vi "save.vi"(8 "error in (no error)":errorcluster, 11 "ScriptEditorV2 in":refnum<class "ScriptEditorV2.lvclass">) -> (0 "error out":errorcluster, 3 "ScriptEditorV2 out":refnum<class "ScriptEditorV2.lvclass">)   [LabVIEW 2009, in "Views.lvlib" / "ScriptEditor.lvlib" / "ScriptEditorV2.lvclass"]
uses:
  ScriptEditorV2.lvclass
  ScriptEditorV2.lvclass/ScriptEditorV2.ctl
  Tools/Scripting/DataPointScript/DataPointScript.lvclass
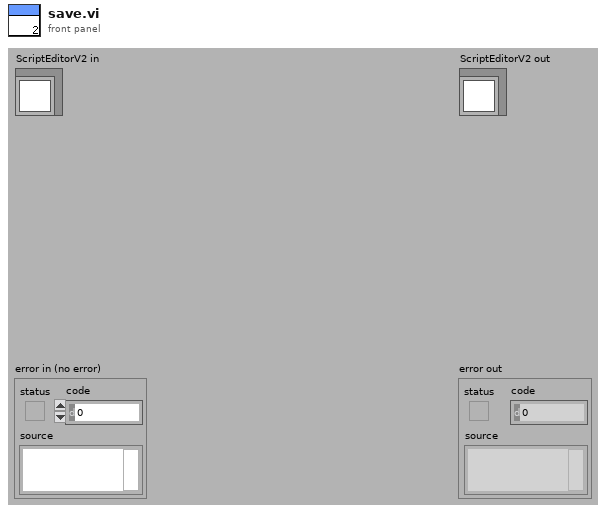
[diagram p1: front panel]
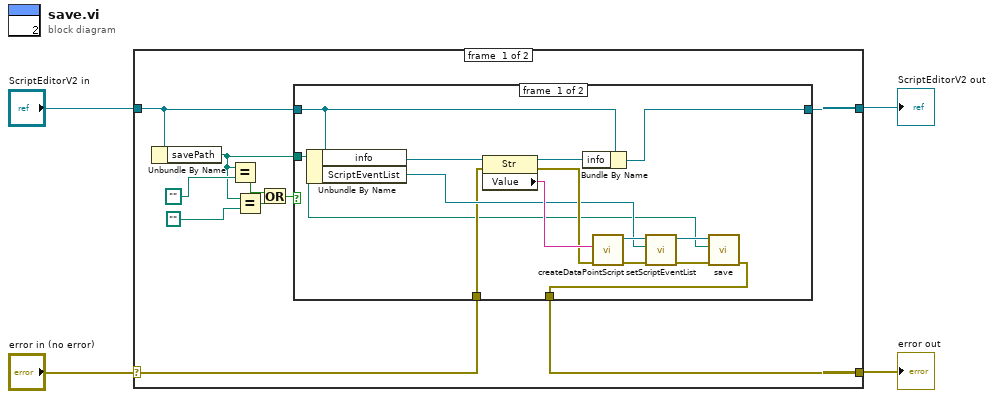
[diagram p0: block diagram]
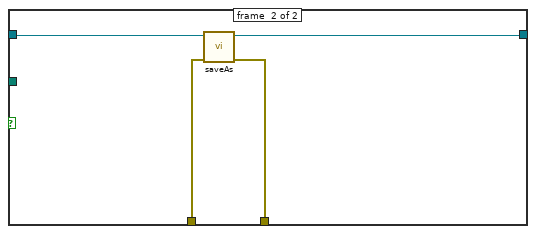
[diagram p2: hidden frame]
diagram:
  n1 = case shown="No Error" "error in (no error)" {
    selector: "error in (no error)" -> [w12 w34]
    tunnel: [w13 w34] -> w3
    tunnel: [w14 w33] -> w1
    tunnel: "ScriptEditorV2 in" -> [w11 w33]
    frame #0 {
      n2 = Unbundle By Name(w11) -> ("savePath"=w5:path)
      n3 = Equal?(x=w5, y=path "") -> (x = y?=w10:bool)
      n4 = Equal?(x=w5, y=path "") -> (x = y?=w7:bool)
      n5 = Or(x=w10, y=w7) -> (x .or. y?=w6:bool)
      n6 = case shown="False" w6 {
        tunnel: w11 -> [w24 w32]
        tunnel: [w23 w29] -> w14
        tunnel: [w17 w30] -> w13
        tunnel: w12 -> [w16 w31]
        tunnel: w5 -> [w15 _]
        frame #0 {
          n7 = Unbundle By Name(w24) -> ("info"=w28:refnum<vi>, "ScriptEventList"=w20:refnum<class "ScriptEventList.lvclass">)
          n8 = property class="Str"(reference=w28, error in=w16) -> (reference out=w25:refnum<vi>, error out=w26:errorcluster, "Value"=w27:string)
          n9 = Bundle By Name(cluster=w24, "info"=w25) -> (w23:refnum<class "ScriptEditorV2.lvclass">)
          n10 = call "createDataPointScript.vi"("error in (no error)"=w26, "script_comment"=w27) -> ("error out"=w22:errorcluster, "DataPointScript out"=w21:refnum<class "DataPointScript.lvclass">)  [unwired: 8 in]
          n11 = call "setScriptEventList.vi"("error in (no error)"=w22, "TScriptEventList"=w20, "DataPointScript.lvclass in"=w21) -> ("error out"=w19:errorcluster, "DataPointScript.lvclass out"=w18:refnum<class "DataPointScript.lvclass">)  [unwired: 7 in]
          n12 = call "save.vi"("error in (no error)"=w19, "Path"=w15, "DataPointScript in"=w18) -> ("error out"=w17:errorcluster)  [unwired: 7 in, 1 out]
        }
        frame #1 {
          n13 = call "saveAs.vi"("error in (no error)"=w31, "ScriptEditorV2 in"=w32) -> ("error out"=w30:errorcluster, "ScriptEditorV2 out"=w29:refnum<class "ScriptEditorV2.lvclass">)  [unwired: 8 in]
        }
      }
    }
    frame #1 {
    }
  }
  "error out" <- w3
  "ScriptEditorV2 out" <- w1
